vi "PSVCH_Check.vi"(8 "Error In (no error)":errorcluster, 10 "VarList":T1, 11 "Formula":string) -> (0 "Error Out":errorcluster, 2 "source":string, 3 "code":i32)   [LabVIEW 2016]
panel:
  # "Data In"
  # "Data Out"
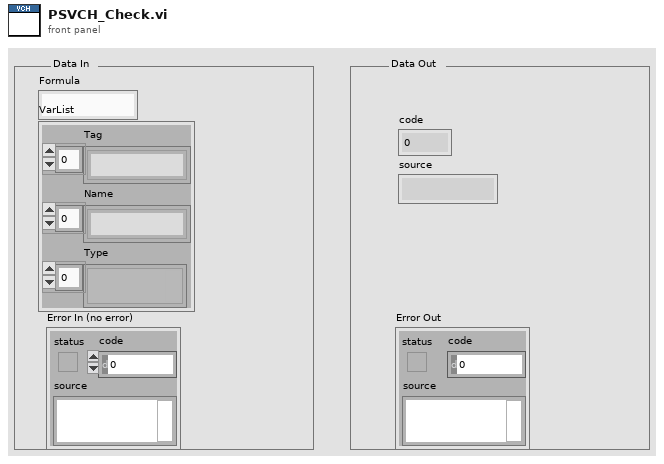
[diagram p1: front panel]
types:
  T1 = cluster{"Tag":string[], "Name":string[], "Type":variant[]}
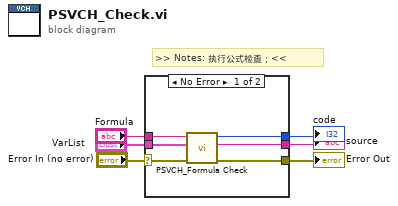
[diagram p0: block diagram]
diagram:
  # ">> Notes: 执行公式检查；<<"
  n1 = case shown="No Error" "Error In (no error)" {
    selector: "Error In (no error)" -> [w12 w13]
    tunnel: [w10 w13] -> w5
    tunnel: "Formula" -> [w11 _]
    tunnel: [w9 _] -> w3
    tunnel: [w8 _] -> w2
    tunnel: "VarList" -> [w7 _]
    frame No Error {
      n2 = call "PSVCH_Formula Check.vi"("Error In (no error)"=w12, "VarList"=w7, "Formula"=w11) -> ("Error Out"=w10:errorcluster, "source"=w8:string, "code"=w9:i32)  [unwired: 4 in, 2 out]
    }
    frame Error {
    }
  }
  "Error Out" <- w5
  "code" <- w3
  "source" <- w2
